vi "Calibrate Fish Shaker.vi"() -> ()   [LabVIEW 2015]
uses:
  Type Defs/Cal Stimulus.ctl
  Utility VIs/Conversion VIs/Create Waveform Cluster (2D).vi
  Utility VIs/Math VIs/FFT x(t) to dB,Degrees (2D).vi
  Instance           1 24Saved   Calibrate In Ear .vi
panel:
  in  "Gain (dB)":dbl
  out "start signal":bool
  out "exit signal":bool
  in  "Plot max acceleration":bool=TRUE
  in  "Load":bool
  in  "Clear":bool
  in  "Accelerometer sens":dbl caption="Accelerometer \nsensitivity \n(mV/g)"
  out "Path":path
  out "Acquired":i32=256
  in  "Stimulus":T1={"Min Freq (Hz)"=1000.0, "Max Freq (Hz)"=50000.0, "Freq Step (Hz)"=50.0, "Waveform"=enum."Chirp", "Attenuation (dB)"=30.0, "Sample Rate (Hz)"=100000.0}
  out "ASTF phase":cluster{"Frequency":dbl[], "Frequency":dbl[]}[](graph)
  out "ASTF mag":cluster{"Frequency":dbl[], "Frequency":dbl[]}[](graph)
  out "Mic phase graph":cluster{"offset":dbl, "dx":dbl, "Y":dbl[][]}(graph)
  out "Mic mag graph":cluster{"offset":dbl, "dx":dbl, "Y":dbl[][]}(graph)
  out "Mic signals":cluster{"offset":dbl, "dx":dbl, "Y":dbl[][]}(graph)
  out "Stimulus graph":cluster{i32, dbl, dbl[]}(graph)={0, 0.01, []}
  in  "Averages":i32=128
  in  "RETURN":bool
  in  "START":bool
  in  "STOP":bool
  # "Raw Data"
  # "Shaker Transfer Function"
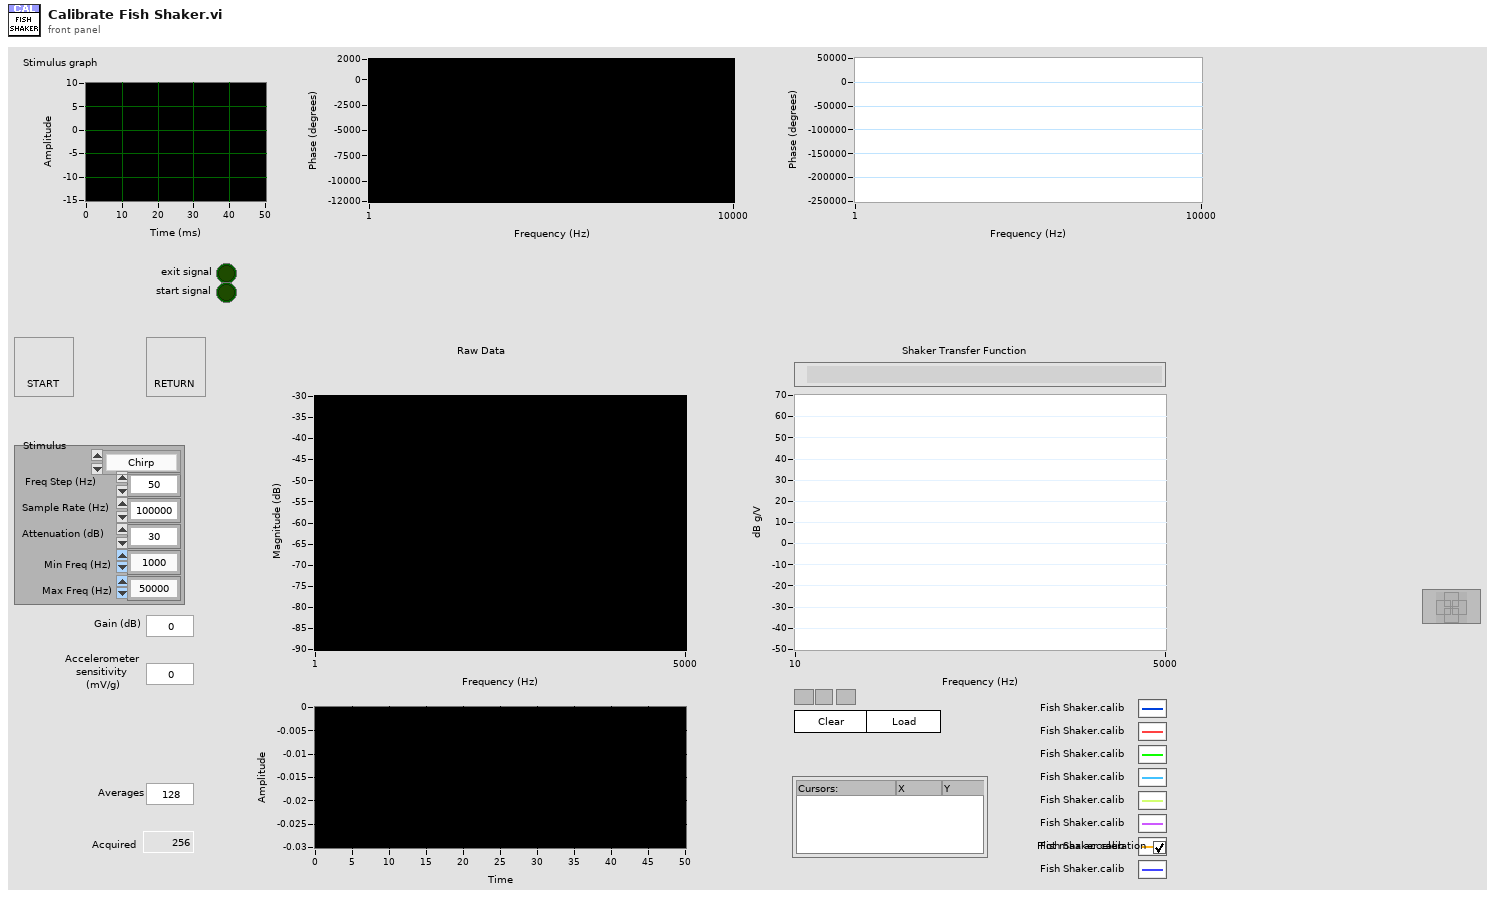
[diagram p1: front panel]
types:
  T1 = typedef "Cal Stimulus.ctl" = cluster{"Min Freq (Hz)":dbl, "Max Freq (Hz)":dbl, "Freq Step (Hz)":dbl, "Waveform":enum16{"Chirp", "Weighted"}, "Attenuation (dB)":dbl, "Sample Rate (Hz)":dbl}
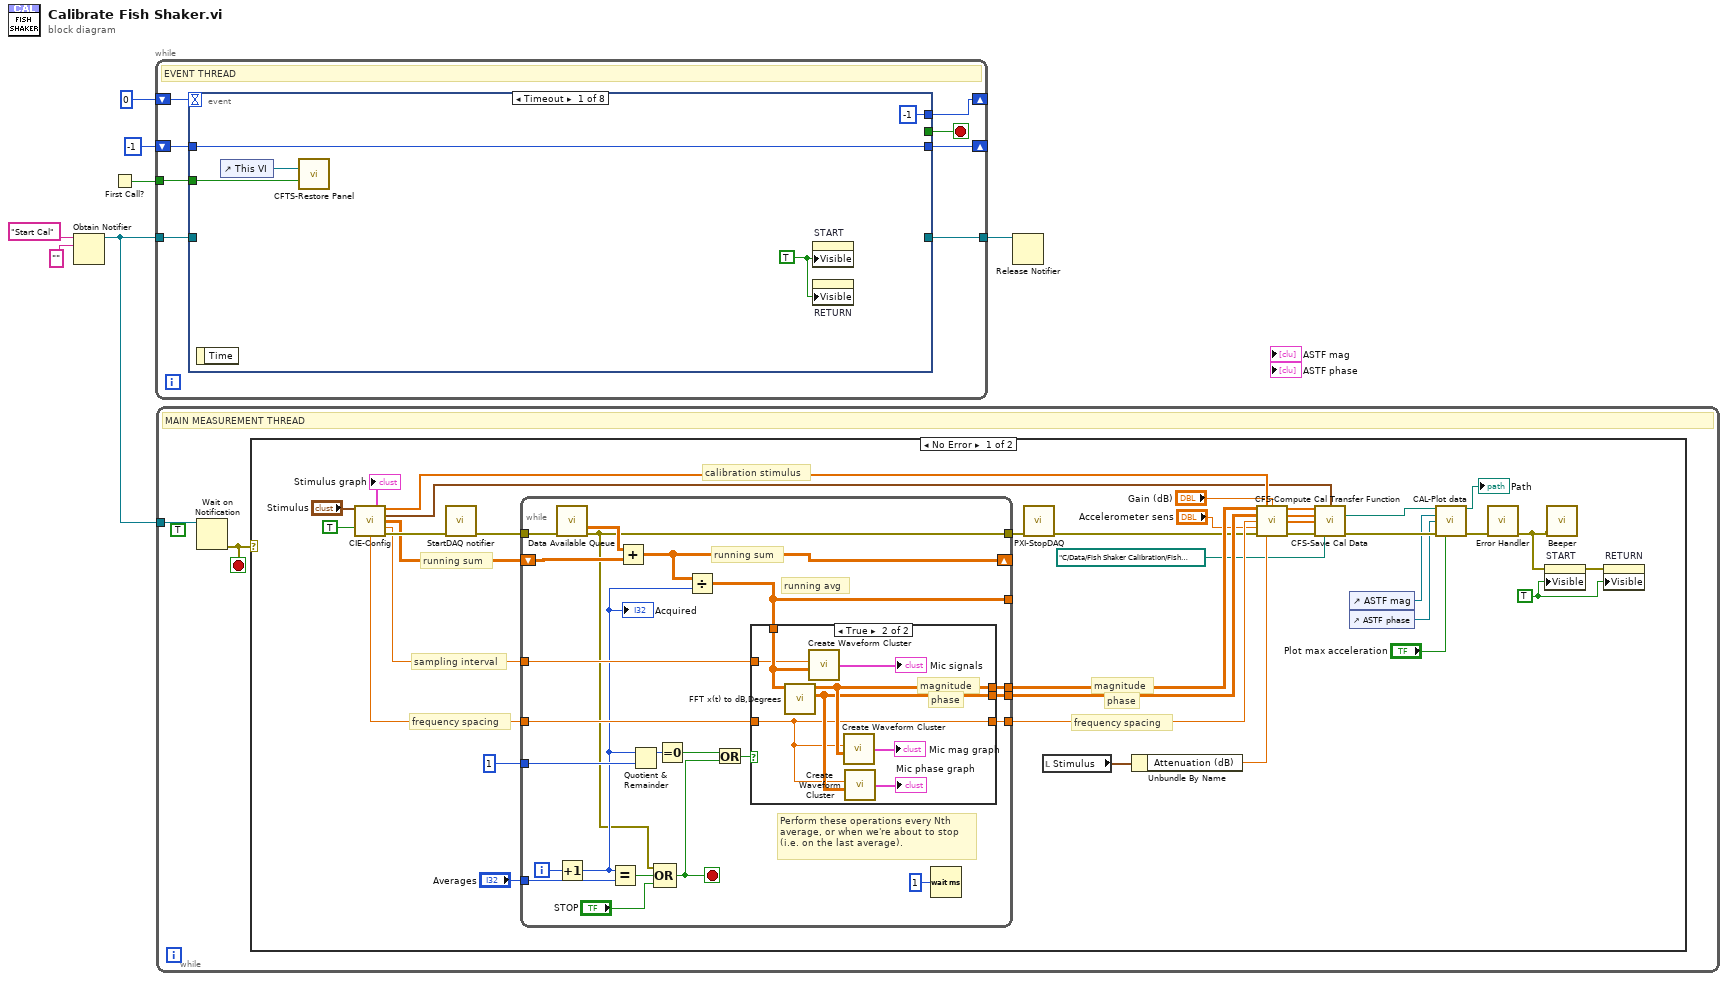
[diagram p0: block diagram]
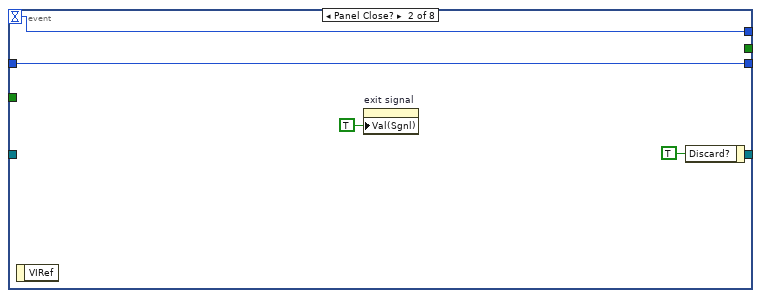
[diagram p4: hidden frame]
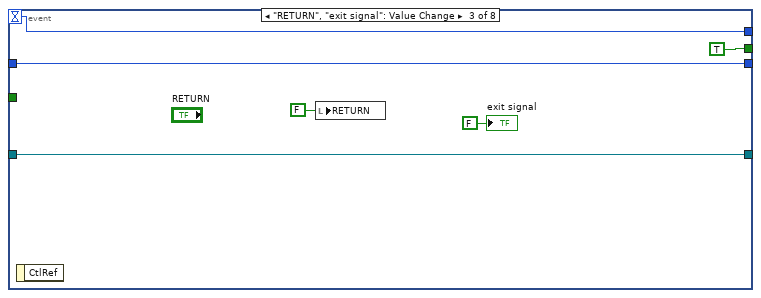
[diagram p5: hidden frame]
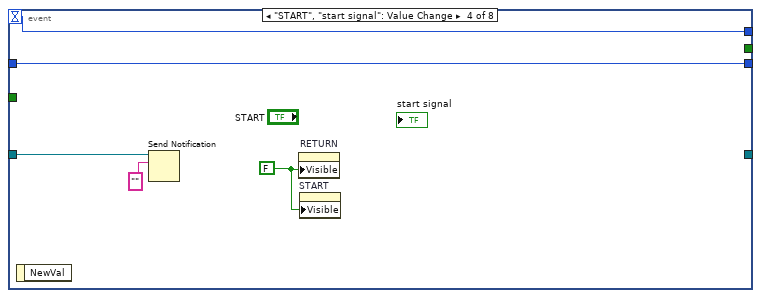
[diagram p6: hidden frame]
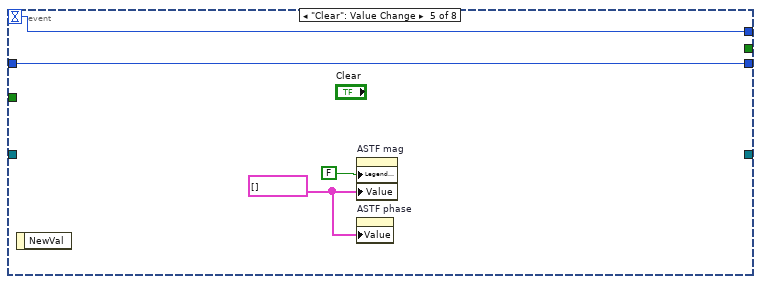
[diagram p7: hidden frame]
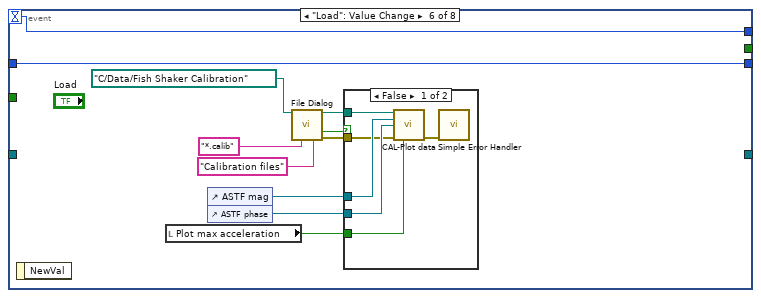
[diagram p8: hidden frame]
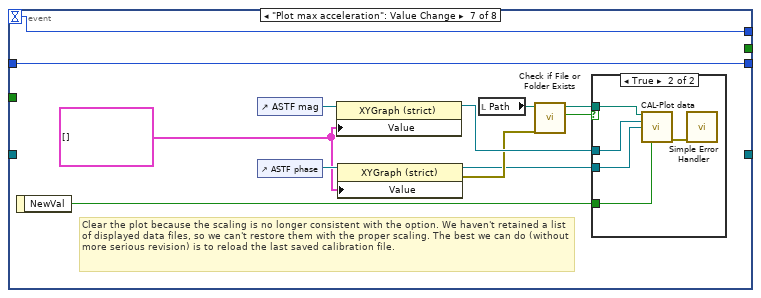
[diagram p10: hidden frame]
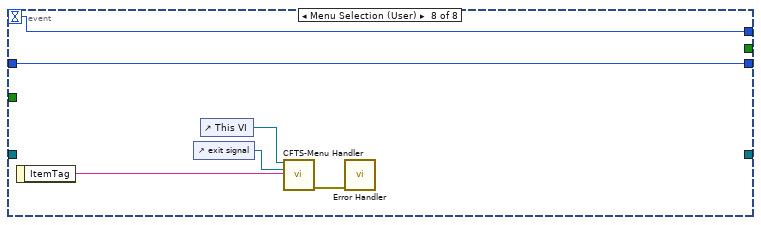
[diagram p12: hidden frame]
diagram:
  n1 = Obtain Notifier(name (unnamed)="Start Cal", notification data type="") -> (notifier out=w7:refnum<notifier>)  [unwired: 2 in, 2 out]
  n2 = First Call?() -> (First Call?: T/F=w2:bool)
  n3 = while {
    tunnel: w7 -> [w14]
    tunnel: [w13] -> w6
    shift-right: [w11] -> _
    shift-left: 0 -> [w12]
    tunnel: w2 -> [w10]
    shift-right: [w8] -> _
    shift-left: -1 -> [w9]
    stop <- w15 stop-if-true
    # "EVENT THREAD"
    n4 = event shown="[0] Timeout" {
      selector: _ -> [_ _ _ _ _ _ _ _]
      dyn-events: _ -> [_ _ _ _ _ _ _ _]
      timeout: w12 -> [_ w24 w28 w34 w37 w43 w68 w79]
      tunnel: [_ _ TRUE _ _ _ _ _] -> w15
      tunnel: w14 -> [_ _ w29 w35 _ _ _ _]
      tunnel: [_ _ w29 _ _ _ _ _] -> w13
      tunnel: [-1 w24 w28 w34 w37 w43 w68 w79] -> w11
      tunnel: w10 -> [w17 _ _ _ _ _ _ _]
      tunnel: w9 -> [w16 w21 w25 w31 w36 w41 w57 w74]
      tunnel: [w16 w21 w25 w31 w36 w41 w57 w74] -> w8
      event Timeout {
        w19 = TRUE ("Visible")
        n5 = event-data() -> ()  [unwired: 1 in, 1 out]
        n6 = control-ref of="This VI"() -> (w18:refnum<vi>)
        n7 = call "CFTS-Restore Panel.vi"("VI refnum"=w18, "Restore?"=w17) -> ()  [unwired: 12 in, 2 out]
        n8 = property on="START" class="Bool"("Visible"=w19) -> ()  [unwired: 2 in, 2 out]
        n9 = property on="RETURN" class="Bool (strict)"("Visible"=w19) -> ()  [unwired: 2 in, 2 out]
      }
      event Panel Close? {
        n10 = event-data() -> ()  [unwired: 1 in, 1 out]
        n11 = property on="exit signal" class="Bool (strict)"("Val(Sgnl)"=TRUE ("Value (Signaling)")) -> ()  [unwired: 2 in, 2 out]
        n12 = event-data("Discard?"=TRUE) -> ()  [unwired: 1 in, 1 out]
      }
      event "RETURN", "exit signal": Value Change {
        n13 = event-data() -> ()  [unwired: 1 in, 1 out]
        n14 = local write "RETURN"(FALSE ("RETURN")) -> ()
        "exit signal" <- FALSE ("exit signal")
      }
      event "START", "start signal": Value Change {
        w32 = FALSE
        n15 = event-data() -> ()  [unwired: 1 in, 1 out]
        n16 = Send Notification(notification="", notifier=w35) -> ()  [unwired: 1 in, 2 out]
        n17 = property on="RETURN" class="Bool (strict)"("Visible"=w32) -> ()  [unwired: 2 in, 2 out]
        n18 = property on="START" class="Bool"("Visible"=w32) -> ()  [unwired: 2 in, 2 out]
      }
      event "Clear": Value Change {
        w38 = cluster{"Frequency":dbl[], "Frequency":dbl[]}[] [] ("ASTF mag")
        n19 = event-data() -> ()  [unwired: 1 in, 1 out]
        n20 = property on="ASTF mag" class="XYGraph (strict)"("Legend Visible"=FALSE ("Legend:Visible"), "Value"=w38) -> ()  [unwired: 2 in, 2 out]
        n21 = property on="ASTF phase" class="XYGraph (strict)"("Value"=w38) -> ()  [unwired: 2 in, 2 out]
      }
      event "Load": Value Change {
        n22 = event-data() -> ()  [unwired: 1 in, 1 out]
        n23 = local read "Plot max acceleration"() -> (w42:bool)
        n24 = control-ref of="ASTF mag"() -> (w48:refnum<vi>)
        n25 = control-ref of="ASTF phase"() -> (w47:refnum<vi>)
        n26 = call "File Dialog"("start path"=path "C:/Data/Fish Shaker Calibration" ("appended path"), "pattern (all files)"="*.calib", "pattern label"="Calibration files") -> ("selected path"=w50:path, "cancelled"=w49:bool, "error out"=w46:errorcluster)  [unwired: 9 in, 1 out]
        n27 = case shown="False" w49 {
          tunnel: w50 -> [w56 _]
          tunnel: w48 -> [w55 _]
          tunnel: w47 -> [w54 _]
          tunnel: w46 -> [w52 _]
          tunnel: w42 -> [w51 _]
          frame False {
            n28 = call "CAL-Plot data.vi"("Path"=w56, "Mag graph"=w55, "Phase graph"=w54, "error in (no error)"=w52, "Plot Max SPL (F)"=w51) -> ("error out"=w53:errorcluster)  [unwired: 9 in, 1 out]
            n29 = call <vilib>:"Simple Error Handler.vi"("error in (no error)"=w53) -> ()  [unwired: 4 in, 5 out]
          }
          frame True {
          }
        }
      }
      event "Plot max acceleration": Value Change {
        w59 = cluster{"Frequency":dbl[], "Frequency":dbl[]}[] [] ("Value")
        # "Clear the plot because the scaling is no longer consistent with the option. We haven't retained a list of displayed data files, so we can't restore them with the proper scaling. The best we can do (without more serious revision) is to reload the last saved calibration file."
        n30 = event-data() -> ("NewVal"=w64:bool)  [unwired: 1 in]
        n31 = control-ref of="ASTF mag"() -> (w63:refnum<vi>)
        n32 = control-ref of="ASTF phase"() -> (w60:refnum<vi>)
        n33 = property class="XYGraph (strict)"(reference=w63, "Value"=w59) -> (reference out=w62:refnum<vi>)  [unwired: 1 in, 1 out]
        n34 = property class="XYGraph (strict)"(reference=w60, "Value"=w59) -> (reference out=w58:refnum<vi>, error out=w61:errorcluster)  [unwired: 1 in]
        n35 = local read "Path"() -> (w66:path)
        n36 = call <vilib>:"Check if File or Folder Exists.vi"("error in (no error)"=w61, "path"=w66) -> ("file or folder exists?"=w67:bool, "dup path"=w65:path)  [unwired: 7 in, 1 out]
        n37 = case shown="True" w67 {
          tunnel: w62 -> [_ w73]
          tunnel: w58 -> [_ w72]
          tunnel: w64 -> [_ w70]
          tunnel: w65 -> [_ w69]
          frame False {
          }
          frame True {
            n38 = call "CAL-Plot data.vi"("Path"=w69, "Mag graph"=w73, "Phase graph"=w72, "Plot Max SPL (F)"=w70) -> ("error out"=w71:errorcluster)  [unwired: 10 in, 1 out]
            n39 = call <vilib>:"Simple Error Handler.vi"("error in (no error)"=w71) -> ()  [unwired: 4 in, 5 out]
          }
        }
      }
      event Menu Selection (User) {
        n40 = event-data() -> ("ItemTag"=w78:string)  [unwired: 1 in]
        n41 = control-ref of="exit signal"() -> (w75:refnum<vi>)
        n42 = control-ref of="This VI"() -> (w77:refnum<vi>)
        n43 = call "CFTS-Menu Handler.vi"("VI Refnum"=w77, "Return Refnum"=w75, "ItemTag"=w78) -> ("error out"=w76:errorcluster)  [unwired: 11 in, 1 out]
        n44 = call "Error Handler.vi"("error in (no error)"=w76) -> ()  [unwired: 13 in, 2 out]
      }
    }
  }
  n45 = while {
    tunnel: w7 -> [w81]
    stop <- w80 stop-if-true
    (unwired) TRUE
    # "MAIN MEASUREMENT THREAD"
    n46 = Wait on Notification(notifier=w81) -> (error out=w80:errorcluster)  [unwired: 3 in, 3 out]
    n47 = case shown="No Error" w80 {
      frame No Error {
        w87 = TRUE
        # "phase"
        # "magnitude"
        # "frequency spacing"
        # "calibration stimulus"
        # "frequency spacing"
        # "sampling interval"
        # "running sum"
        n48 = call "CIE-Config.vi"("Cal Stimulus"="Stimulus", "Fish shaker"=TRUE) -> ("Stimulus waveform"=→"Stimulus graph":cluster{i32, dbl, dbl[]}, "Stimulus"=w110:dbl[], "Cal Spec Out"=w93:T1, "Mic Avg"=w116:dbl[][], "dt (ms)"=w114:dbl, "df (Hz)"=w115:dbl, "error out"=w117:errorcluster)  [unwired: 7 in]
        n49 = call "StartDAQ notifier.vi"("error in (no error)"=w117) -> ("error out"=w106:errorcluster)  [unwired: 6 in]
        n50 = while {
          tunnel: w106 -> [w139]
          tunnel: [w120] -> w105
          tunnel: "Averages" -> [w136]
          shift-right: [w134] -> _
          shift-left: w116 -> [w135]
          tunnel: 1 -> [w133]
          tunnel: w115 -> [w128]
          tunnel: [w127] -> w113
          tunnel: [w126] -> w112
          tunnel: w114 -> [w125]
          tunnel: [w124] -> w111
          tunnel: [w118] -> _
          i -> [w138]
          stop <- w129 stop-if-true
          # "Perform these operations every Nth\naverage, or when we're about to stop\n(i.e. on the last average)."
          # "running avg"
          # "running sum"
          n51 = call "Data Available Queue.vi"("error in (no error)"=w139) -> ("AI Waveforms"=w122:dbl[][], "error out"=w120:errorcluster)  [unwired: 10 in, 3 out]
          n52 = Increment(x=w138) -> (x+1=w123:i32)
          "Acquired" <- w123
          n53 = Equal?(x=w123, y=w136) -> (x = y?=w137:bool)
          n54 = Add(x=w122, y=w135) -> (x+y=w134:dbl[][])
          n55 = Quotient & Remainder(x=w123, y=w133) -> (x-y*floor(x/y)=w132:i32)  [unwired: 1 out]
          n56 = Compound Arithmetic op=OR(w120, w137, "STOP") -> (w129:bool)
          n57 = Equal To 0?(x=w132) -> (x = 0?=w130:bool)
          n58 = Divide(x=w134, y=w123) -> (x/y=w118:dbl[][])
          n59 = Or(x=w130, y=w129) -> (x .or. y?=w131:bool)
          n60 = case shown="True" w131 {
            tunnel: w118 -> [_ w143]
            tunnel: w128 -> [_ w140]
            tunnel: [_ w145] -> w127
            tunnel: [_ w144] -> w126
            tunnel: w125 -> [_ w142]
            tunnel: [_ w140] -> w124
            frame False {
            }
            frame True {
              # "phase"
              # "magnitude"
              n61 = call-poly "FFT x(t) to dB,Degrees.vi"("X(t)"=w143) -> ("+Freq Phase of FFT (degrees)"=w144:dbl[][], "+Freq. Mag of FFT (dB rms)"=w145:dbl[][])  [unwired: 9 in]
              n62 = call-poly "Create Waveform Cluster.vi"("dx"=w142, "Array"=w143) -> ("waveform cluster"=→"Mic signals":cluster{"offset":dbl, "dx":dbl, "Y":dbl[][]})  [unwired: 3 in]
              n63 = call-poly "Create Waveform Cluster.vi"("dx"=w140, "Array"=w145) -> ("waveform cluster"=→"Mic mag graph":cluster{"offset":dbl, "dx":dbl, "Y":dbl[][]})  [unwired: 3 in]
              n64 = call-poly "Create Waveform Cluster.vi"("dx"=w140, "Array"=w144) -> ("waveform cluster"=→"Mic phase graph":cluster{"offset":dbl, "dx":dbl, "Y":dbl[][]})  [unwired: 3 in]
            }
          }
          n65 = Wait (ms)(milliseconds to wait=u32 1) -> ()  [unwired: 1 out]
        }
        n66 = call "PXI-StopDAQ.vi"("error in (no error)"=w105) -> ("error out"=w94:errorcluster)  [unwired: 6 in]
        n67 = local read "Stimulus"() -> (w109:T1)
        n68 = Unbundle By Name(w109) -> ("Attenuation (dB)"=w101:dbl)
        n69 = call "CFS-Compute Cal Transfer Function.vi"("Mag"=w113, "Stimulus"=w110, "Accel Gain (dB)"="Gain (dB)", "Phase"=w112, "df (Hz)"=w111, "Accelerometer Sens (mV/g)"="Accelerometer sens", "error in (no error)"=w94, "Attenuation (dB)"=w101) -> ("Mag"=w90:dbl[], "Phase"=w89:dbl[], "Frequency"=w88:dbl[], "error out"=w91:errorcluster)  [unwired: 4 in]
        n70 = call "CFS-Save Cal Data.vi"("Mag"=w90, "Cal Stimulus"=w93, "Phase"=w89, "Frequency"=w88, "error in (no error)"=w91, "path"=path "C:/Data/Fish Shaker Calibration/Fish Shaker.calib" ("appended path")) -> ("new file path"=w99:path, "error out"=w100:errorcluster)  [unwired: 8 in]
        n71 = control-ref of="ASTF mag"() -> (w97:refnum<vi>)
        n72 = control-ref of="ASTF phase"() -> (w96:refnum<vi>)
        n73 = call "CAL-Plot data.vi"("Path"=w99, "Mag graph"=w97, "Phase graph"=w96, "error in (no error)"=w100, "Plot Max SPL (F)"="Plot max acceleration") -> ("Path (out)"=→"Path":path, "error out"=w85:errorcluster)  [unwired: 9 in]
        n74 = call "Error Handler.vi"("error in (no error)"=w85) -> ("No Error"=w84:errorcluster)  [unwired: 13 in, 1 out]
        n75 = property on="START" class="Bool"(error in=w84, "Visible"=w87) -> (error out=w86:errorcluster)  [unwired: 1 in, 1 out]
        n76 = call "Beeper.vi"("error in (no error)"=w84) -> ()  [unwired: 4 in, 1 out]
        n77 = property on="RETURN" class="Bool (strict)"(error in=w86, "Visible"=w87) -> ()  [unwired: 1 in, 2 out]
      }
      frame Error {
      }
    }
  }
  n78 = Release Notifier(notifier=w6) -> ()  [unwired: 2 in, 3 out]
